vi "Cal4-GetCalDataFrFile.vi"(9 "StringName":string, 10 "FileExists?":bool, 11 "CalibFilePath":path) -> (1 "CalibData":string, 2 "HasData":bool)   [LabVIEW 2016]
uses:
  Anemometry Sub Vis/Globals/Calib_global.vi
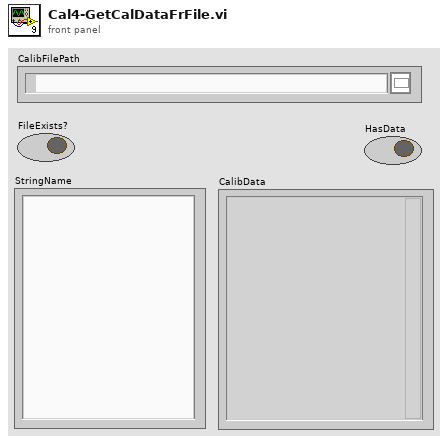
[diagram p1: front panel]
types:
  T1 = typedef "Cal_Inst_type.ctl" = enum16{"Propeller anemometer", "Pressure Transducer", "Hot wire", "Cross wire velocity", "Cross wire angle", "Generic Linear", "Generic Polynomial", "Generic BackPoly", "Fast FID", "Thermocouple", "Cold wire", "Pulsed Wire"}
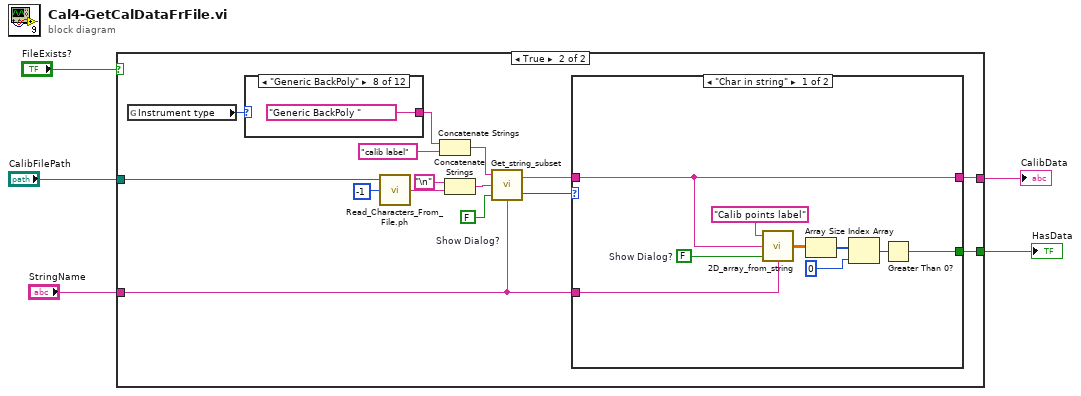
[diagram p0: block diagram]
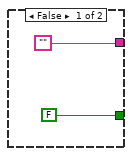
[diagram p2: hidden frame]
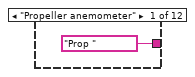
[diagram p3: hidden frame]
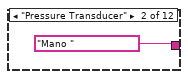
[diagram p4: hidden frame]
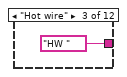
[diagram p5: hidden frame]
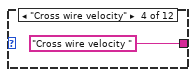
[diagram p6: hidden frame]
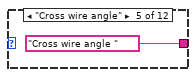
[diagram p7: hidden frame]
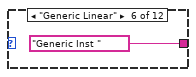
[diagram p8: hidden frame]
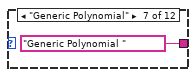
[diagram p9: hidden frame]
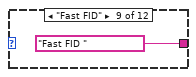
[diagram p10: hidden frame]
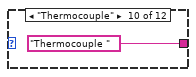
[diagram p11: hidden frame]
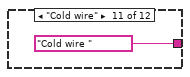
[diagram p12: hidden frame]
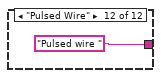
[diagram p13: hidden frame]
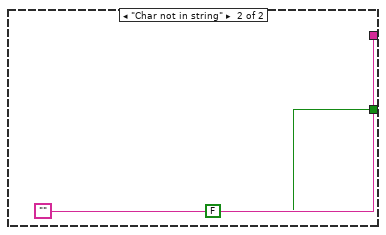
[diagram p14: hidden frame]
diagram:
  n1 = case shown="True" "FileExists?" {
    tunnel: ["" ("Output string") w22] -> w1
    tunnel: [FALSE w21] -> w2
    tunnel: "CalibFilePath" -> [_ w13]
    tunnel: "StringName" -> [_ w8]
    frame False {
    }
    frame True {
      w12 = FALSE  # Show Dialog?
      n2 = global read "Calib_global.vi" "Instrument type"() -> (w16:T1)
      n3 = case shown="\"Generic BackPoly\"" w16 {
        tunnel: ["Prop " "Mano " "HW " "Cross wire velocity " "Cross wire angle " "Generic Inst " "Generic Polynomial " "Generic BackPoly " "Fast FID " "Thermocouple " "Cold wire " "Pulsed wire "] -> w17
        frame "Propeller anemometer" {
        }
        frame "Pressure Transducer" {
        }
        frame "Hot wire" {
        }
        frame "Cross wire velocity" {
        }
        frame "Cross wire angle" {
        }
        frame "Generic Linear" {
        }
        frame "Generic Polynomial" {
        }
        frame "Generic BackPoly" {
        }
        frame "Fast FID" {
        }
        frame "Thermocouple" {
        }
        frame "Cold wire" {
        }
        frame "Pulsed Wire" {
        }
      }
      n4 = call "Read_Characters_From_File.ph.vi"("file path (dialog if empty)"=w13, "number of characters (all:-1)"=-1) -> ("character string"=w10:string)  [unwired: 7 out]
      n5 = Concatenate Strings(w17, "calib label") -> (w18:string)
      n6 = Concatenate Strings("\n", w10) -> (w9:string)
      n7 = call "Get_string_subset.vi"("String Name"=w8, "Show Dialog?"=w12, "String to split"=w9, "File Label"=w18) -> ("Status"=w15:enum16{"Char in string", "Char not in string"}, "Output string"=w14:string)
      n8 = case shown="\"Char in string\"" w15 {
        tunnel: w14 -> [w41 _]
        tunnel: [w41 ""] -> w22
        tunnel: [w36 FALSE] -> w21
        tunnel: w8 -> [w35 _]
        frame "Char in string" {
          w42 = FALSE  # Show Dialog?
          n9 = call "2D_array_from_string.vi"("String Name"=w35, "Show Dialog?"=w42, "Input string"=w41, "Array title"="Calib points label") -> ("2D data array"=w40:dbl[][])
          n10 = Array Size(array=w40) -> (size(s)=w39:i32[])
          n11 = Index Array(array=w39, index=0 ("Index")) -> (element=w37:i32)
          n12 = Greater Than 0?(x=w37) -> (x > 0?=w36:bool)
        }
        frame "Char not in string" {
        }
      }
    }
  }
  "HasData" <- w2
  "CalibData" <- w1
